vi "Build CVT.vi"(8 "Error In":errorcluster, 11 "Controller in":refnum<class "Controller.lvclass">) -> (0 "Error Out":errorcluster, 3 "Controller out":refnum<class "Controller.lvclass">)   [LabVIEW 2014, in "Controller.lvlib" / "Controller.lvclass"]
uses:
  Controller.lvclass
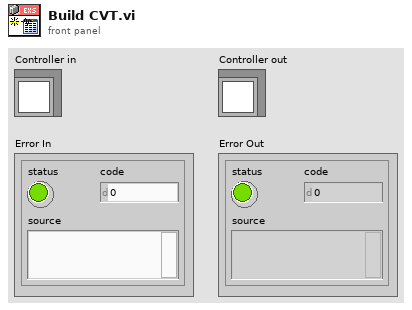
[diagram p1: front panel]
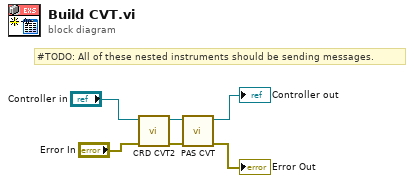
[diagram p0: block diagram]
diagram:
  # "#TODO: All of these nested instruments should be sending messages."
  n1 = call "CRD CVT2.vi"("error in"="Error In", "Controller in"="Controller in") -> ("error out"=w6:errorcluster, "Controller out"=w4:refnum<class "Controller.lvclass">)  [unwired: 8 in]
  n2 = call "PAS CVT.vi"("error in"=w6, "Controller in"=w4) -> ("error out"=→"Error Out":errorcluster, "Controller out"=→"Controller out":refnum<class "Controller.lvclass">)  [unwired: 8 in]
